vi "Update Tree.vi"(8 "error in (no error)":errorcluster, 11 "BuildServer in":refnum<class "BuildServer.lvclass">) -> (0 "error out":errorcluster, 3 "BuildServer out":refnum<class "BuildServer.lvclass">)   [LabVIEW 2017, in "BuildServer.lvlib" / "BuildServer.lvclass"]
uses:
  BuildServer.lvclass
  Classes/Task Interface/Task/Task.lvclass
  BuildServer.lvclass/BuildServer.ctl
  Classes/Task Interface/Task/Task.lvclass/Task.ctl
  Classes/Task Interface/Task/Get Target.vi
  Classes/Task Interface/Task/Read BuildSpec Type.vi
  Classes/Task Interface/Task/Get BuildSpec Name.vi
  Classes/Task Interface/Task/Get ProjectName.vi
  <vilib>/BenjaminR/LookUp Table API/LUT.lvclass
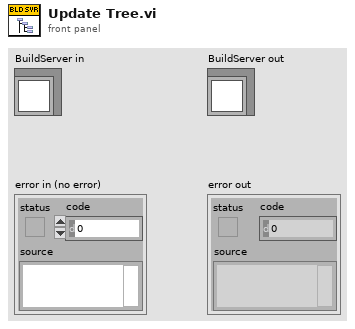
[diagram p1: front panel]
types:
  T1 = typedef "BuildServer.lvlib/BuildServer.lvclass/ProjectOrganization.ctl" = enum16{"Group by Project", "Group by Target", "Group by Type", "Group by Name"}
  T2 = cluster{cluster{"Properties:BuildSpec Name":string, i32}[]}[]
  T3 = cluster{cluster{"Properties:BuildSpec Name":string, i32}[]}
  T4 = cluster{"Properties:BuildSpec Name":string, i32}[]
  T5 = cluster{"Left Cell String":string, "Child Text":string[], "Child Tag":string, "Item Indent":i32, "Child Only?":bool, "Glyph Index":i32}[]
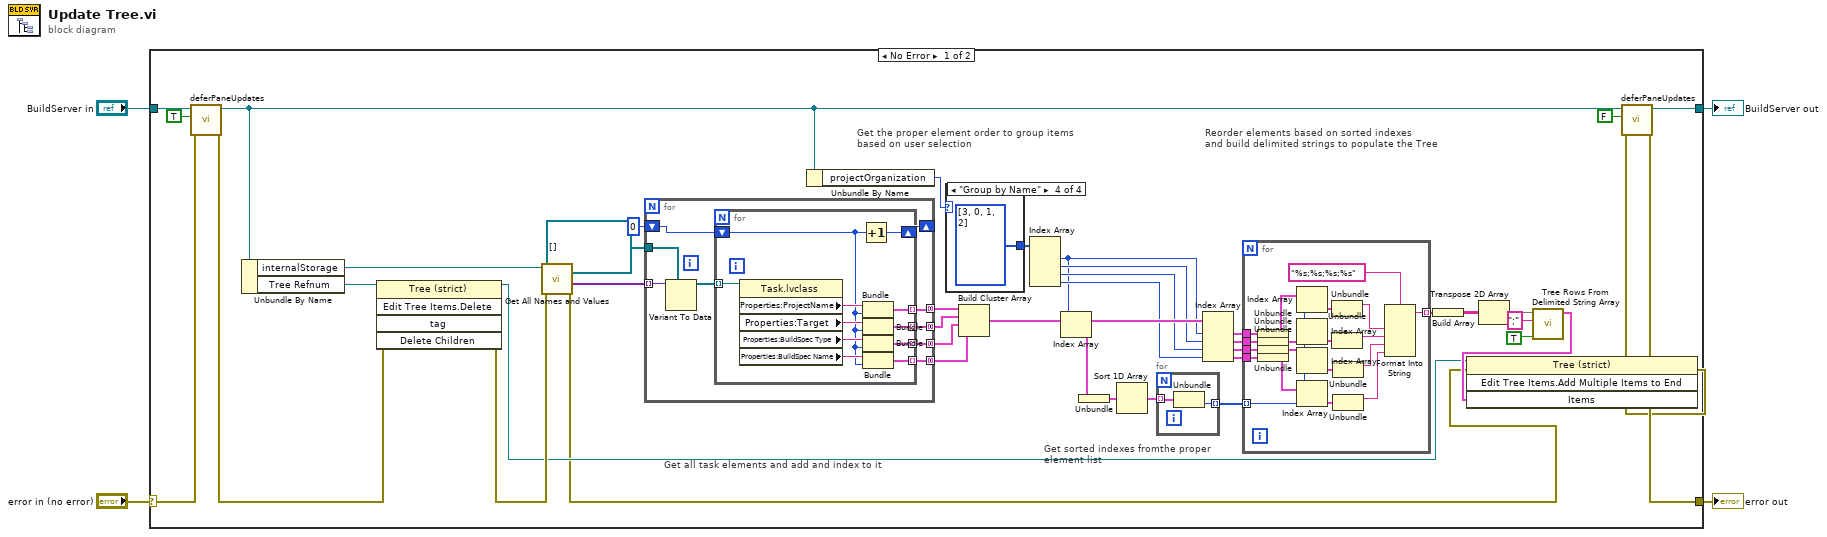
[diagram p0: block diagram]
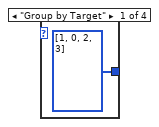
[diagram p2: hidden frame]
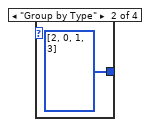
[diagram p3: hidden frame]
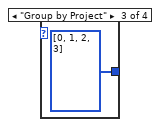
[diagram p4: hidden frame]
diagram:
  n1 = case shown="No Error" "error in (no error)" {
    selector: "error in (no error)" -> [w38 w93]
    tunnel: [w45 w93] -> w3
    tunnel: [w40 w92] -> w1
    tunnel: "BuildServer in" -> [w41 w92]
    frame No Error {
      # "Reorder elements based on sorted indexes\nand build delimited strings to populate the Tree"
      # "Get sorted indexes fromthe proper\nelement list"
      # "Get the proper element order to group items\nbased on user selection"
      # "Get all task elements and add and index to it"
      n2 = call "deferPaneUpdates.vi"("error in (no error)"=w38, "Defer Updates"=TRUE, "BuildServer in"=w41) -> ("error out"=w37:errorcluster, "BuildServer out"=w27:refnum<class "BuildServer.lvclass">)  [unwired: 7 in]
      n3 = Unbundle By Name(w27) -> ("internalStorage"=w44:refnum<class "LUT.lvclass">, "Tree Refnum"=w43:refnum<vi>)
      n4 = invoke class="Tree (strict)" method="Edit Tree Items.Delete"(reference=w43, error in=w37) -> (reference out=w7:refnum<vi>, error out=w42:errorcluster)  [unwired: 3 in, 3 out]
      n5 = call <vilib>:"Get All Names and Values.vi"("error in (no error)"=w42, "LUT in"=w44) -> ("error out"=w6:errorcluster, "Values"=w35:variant[])  [unwired: 6 in, 2 out]
      n6 = for {
        tunnel: w35 -> [w80] mode=indexing
        tunnel: refnum<class "Task.lvclass">[] [] -> [w79]
        tunnel: [w78] -> w28 mode=concatenating
        tunnel: [w77] -> w29 mode=concatenating
        tunnel: [w76] -> w30 mode=concatenating
        tunnel: [w75] -> w31 mode=concatenating
        shift-right: [w73] -> _
        shift-left: 0 -> [w74]
        n7 = Variant To Data(type=w79, Variant=w80) -> (data=w72:refnum<class "Task.lvclass">[])  [unwired: 1 in, 1 out]
        n8 = for {
          tunnel: [w87] -> w75 mode=indexing
          tunnel: [w86] -> w76 mode=indexing
          tunnel: [w85] -> w77 mode=indexing
          tunnel: [w84] -> w78 mode=indexing
          shift-right: [w82] -> w73
          shift-left: w74 -> [w83]
          tunnel: w72 -> [w81] mode=indexing
          n9 = property class="Task.lvclass"(reference=w81) -> ("Properties:ProjectName"=w88:string, "Properties:Target"=w89:string, "Properties:BuildSpec Type"=w90:string, "Properties:BuildSpec Name"=w91:string)  [unwired: 1 in, 2 out]
          n10 = Increment(x=w83) -> (x+1=w82:i32)
          n11 = Bundle("Properties:ProjectName"=w88, w83) -> (w87:cluster{"Properties:ProjectName":string, i32})  [unwired: 1 in]
          n12 = Bundle("Properties:Target"=w89, w83) -> (w86:cluster{"Properties:Target":string, i32})  [unwired: 1 in]
          n13 = Bundle("Properties:BuildSpec Type"=w90, w83) -> (w85:cluster{"Properties:BuildSpec Type":string, i32})  [unwired: 1 in]
          n14 = Bundle("Properties:BuildSpec Name"=w91, w83) -> (w84:cluster{"Properties:BuildSpec Name":string, i32})  [unwired: 1 in]
        }
      }
      n15 = Unbundle By Name(w27) -> ("projectOrganization"=w12:T1)
      n16 = case shown="\"Group by Name\"" w12 {
        tunnel: [i32[] [1, 0, 2, 3] ("index") i32[] [2, 0, 1, 3] ("index") i32[] [0, 1, 2, 3] ("index") i32[] [3, 0, 1, 2] ("index")] -> w23
        frame "Group by Target" {
        }
        frame "Group by Type" {
        }
        frame "Group by Project" {
        }
        frame "Group by Name" {
        }
      }
      n17 = Build Cluster Array(w31, w30, w29, w28) -> (w25:T2)
      n18 = Index Array(array=w23) -> (element #1=w13:i32, element #2=w22:i32, element #3=w21:i32, element #4=w20:i32)  [unwired: 4 in]
      n19 = Index Array(array=w25, index=w13) -> (element=w34:T3)
      n20 = Unbundle(w34) -> (w33:T4)
      n21 = Sort 1D Array(array=w33) -> (sorted array=w32:T4)
      n22 = for {
        tunnel: w32 -> [w71] mode=indexing
        tunnel: [w70] -> w26 mode=indexing
        n23 = Unbundle(w71) -> (w70:i32)  [unwired: 1 out]
      }
      n24 = Index Array(array=w25, index #1=w13, index #2=w22, index #3=w21, index #4=w20) -> (element #1=w24:T3, element #2=w19:T3, element #3=w18:T3, element #4=w17:T3)
      n25 = for {
        tunnel: w26 -> [w58] mode=indexing
        tunnel: w24 -> [w65]
        tunnel: w19 -> [w61]
        tunnel: w18 -> [w60]
        tunnel: w17 -> [w59]
        tunnel: [w47] -> w16 mode=indexing
        n26 = Unbundle(w65) -> (w64:T4)
        n27 = Unbundle(w61) -> (w62:T4)
        n28 = Unbundle(w60) -> (w57:T4)
        n29 = Unbundle(w59) -> (w56:T4)
        n30 = Index Array(array=w64, index=w58) -> (element=w63:cluster{"Properties:BuildSpec Name":string, i32})
        n31 = Index Array(array=w62, index=w58) -> (element=w53:cluster{"Properties:BuildSpec Name":string, i32})
        n32 = Index Array(array=w57, index=w58) -> (element=w54:cluster{"Properties:BuildSpec Name":string, i32})
        n33 = Index Array(array=w56, index=w58) -> (element=w55:cluster{"Properties:BuildSpec Name":string, i32})
        n34 = Unbundle(w63) -> ("Properties:BuildSpec Name"=w52:string)  [unwired: 1 out]
        n35 = Unbundle(w53) -> ("Properties:BuildSpec Name"=w51:string)  [unwired: 1 out]
        n36 = Unbundle(w54) -> ("Properties:BuildSpec Name"=w50:string)  [unwired: 1 out]
        n37 = Unbundle(w55) -> ("Properties:BuildSpec Name"=w49:string)  [unwired: 1 out]
        n38 = Format Into String(format string="%s;%s;%s;%s", w52, w51, w50, w49) -> (resulting string=w47:string)  [unwired: 2 in, 1 out]
      }
      n39 = Build Array(w16) -> (w15:string[][])
      n40 = Transpose 2D Array(2D array=w15) -> (transposed array=w11:string[][])
      n41 = call "Tree Rows From Delimited String Array.vi"("Use Child Only? (False)"=TRUE, "Delimiter"=";", "Items (Delimited)"=w11) -> ("Item to Add[]"=w8:T5)  [unwired: 7 in, 1 out]
      n42 = invoke class="Tree (strict)" method="Edit Tree Items.Add Multiple Items to End"(reference=w7, error in=w6, "Items"=w8) -> (error out=w5:errorcluster)  [unwired: 1 in, 3 out]
      n43 = call "deferPaneUpdates.vi"("error in (no error)"=w5, "Defer Updates"=FALSE, "BuildServer in"=w27) -> ("error out"=w45:errorcluster, "BuildServer out"=w40:refnum<class "BuildServer.lvclass">)  [unwired: 7 in]
    }
    frame Error {
    }
  }
  "error out" <- w3
  "BuildServer out" <- w1
